vi "Close.vi"(8 "error in (no error)":errorcluster, 11 "Interaction By Refererence in":refnum<class "Interaction By Refererence.lvclass">) -> (0 "error out":errorcluster)   [LabVIEW 2013, in "Interaction By Refererence.lvclass"]
uses:
  Interaction By Refererence.lvclass
  Interaction By Refererence.lvclass/Interaction By Refererence.ctl
  IContainer/Interaction/Interaction.lvclass
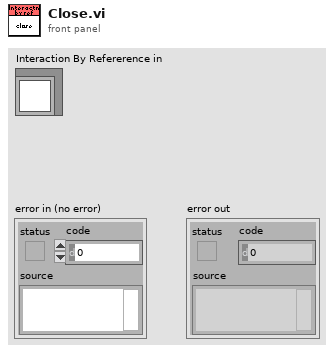
[diagram p1: front panel]
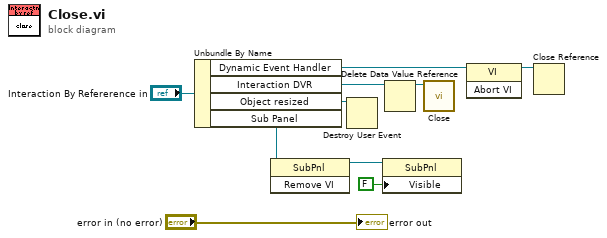
[diagram p0: block diagram]
diagram:
  n1 = Unbundle By Name("Interaction By Refererence in") -> ("Dynamic Event Handler"=w2:refnum<vi>, "Interaction DVR"=w3:refnum<data-value>, "Object resized"=w8:refnum<user-event>, "Sub Panel"=w6:refnum<vi>)
  n2 = invoke class="SubPnl" method="Remove VI"(reference=w6) -> (reference out=w5:refnum<vi>)  [unwired: 2 in, 2 out]
  n3 = Destroy User Event(user event=w8) -> ()  [unwired: 1 in, 1 out]
  n4 = property class="SubPnl"(reference=w5, "Visible"=FALSE) -> ()  [unwired: 1 in, 2 out]
  n5 = Delete Data Value Reference(data value reference=w3) -> (data value=w7:refnum<class "Interaction.lvclass">)  [unwired: 1 in, 1 out]
  n6 = call-dynamic "Close.vi"("Interaction in"=w7) -> ()  [unwired: 10 in, 1 out]
  n7 = invoke class="VI" method="Abort VI"(reference=w2) -> (reference out=w1:refnum<vi>)  [unwired: 2 in, 2 out]
  n8 = Close Reference(reference=w1) -> ()  [unwired: 1 in, 1 out]
  "error out" <- "error in (no error)"
